vi "PV_DataLog_v2.vi"() -> ()   [LabVIEW 2016]
uses:
  MGCC_DataLog_global.vi
  Global tdms reference.vi
  Communication/Global communication.vi
  <vilib>/Utility/error.llb/Error Cluster From Error Code.vi
  Finite State Machine (He Yin)/Sub-VIs/MGCC_FntStaMach_gobal.vi
  <vilib>/ErrorRing/Error Ring.xnode
panel:
  in  "Start":bool=TRUE
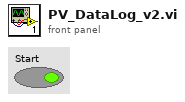
[diagram p1: front panel]
types:
  T1 = enum16{"open", "open or create", "create or replace", "create", "open (read-only)"}
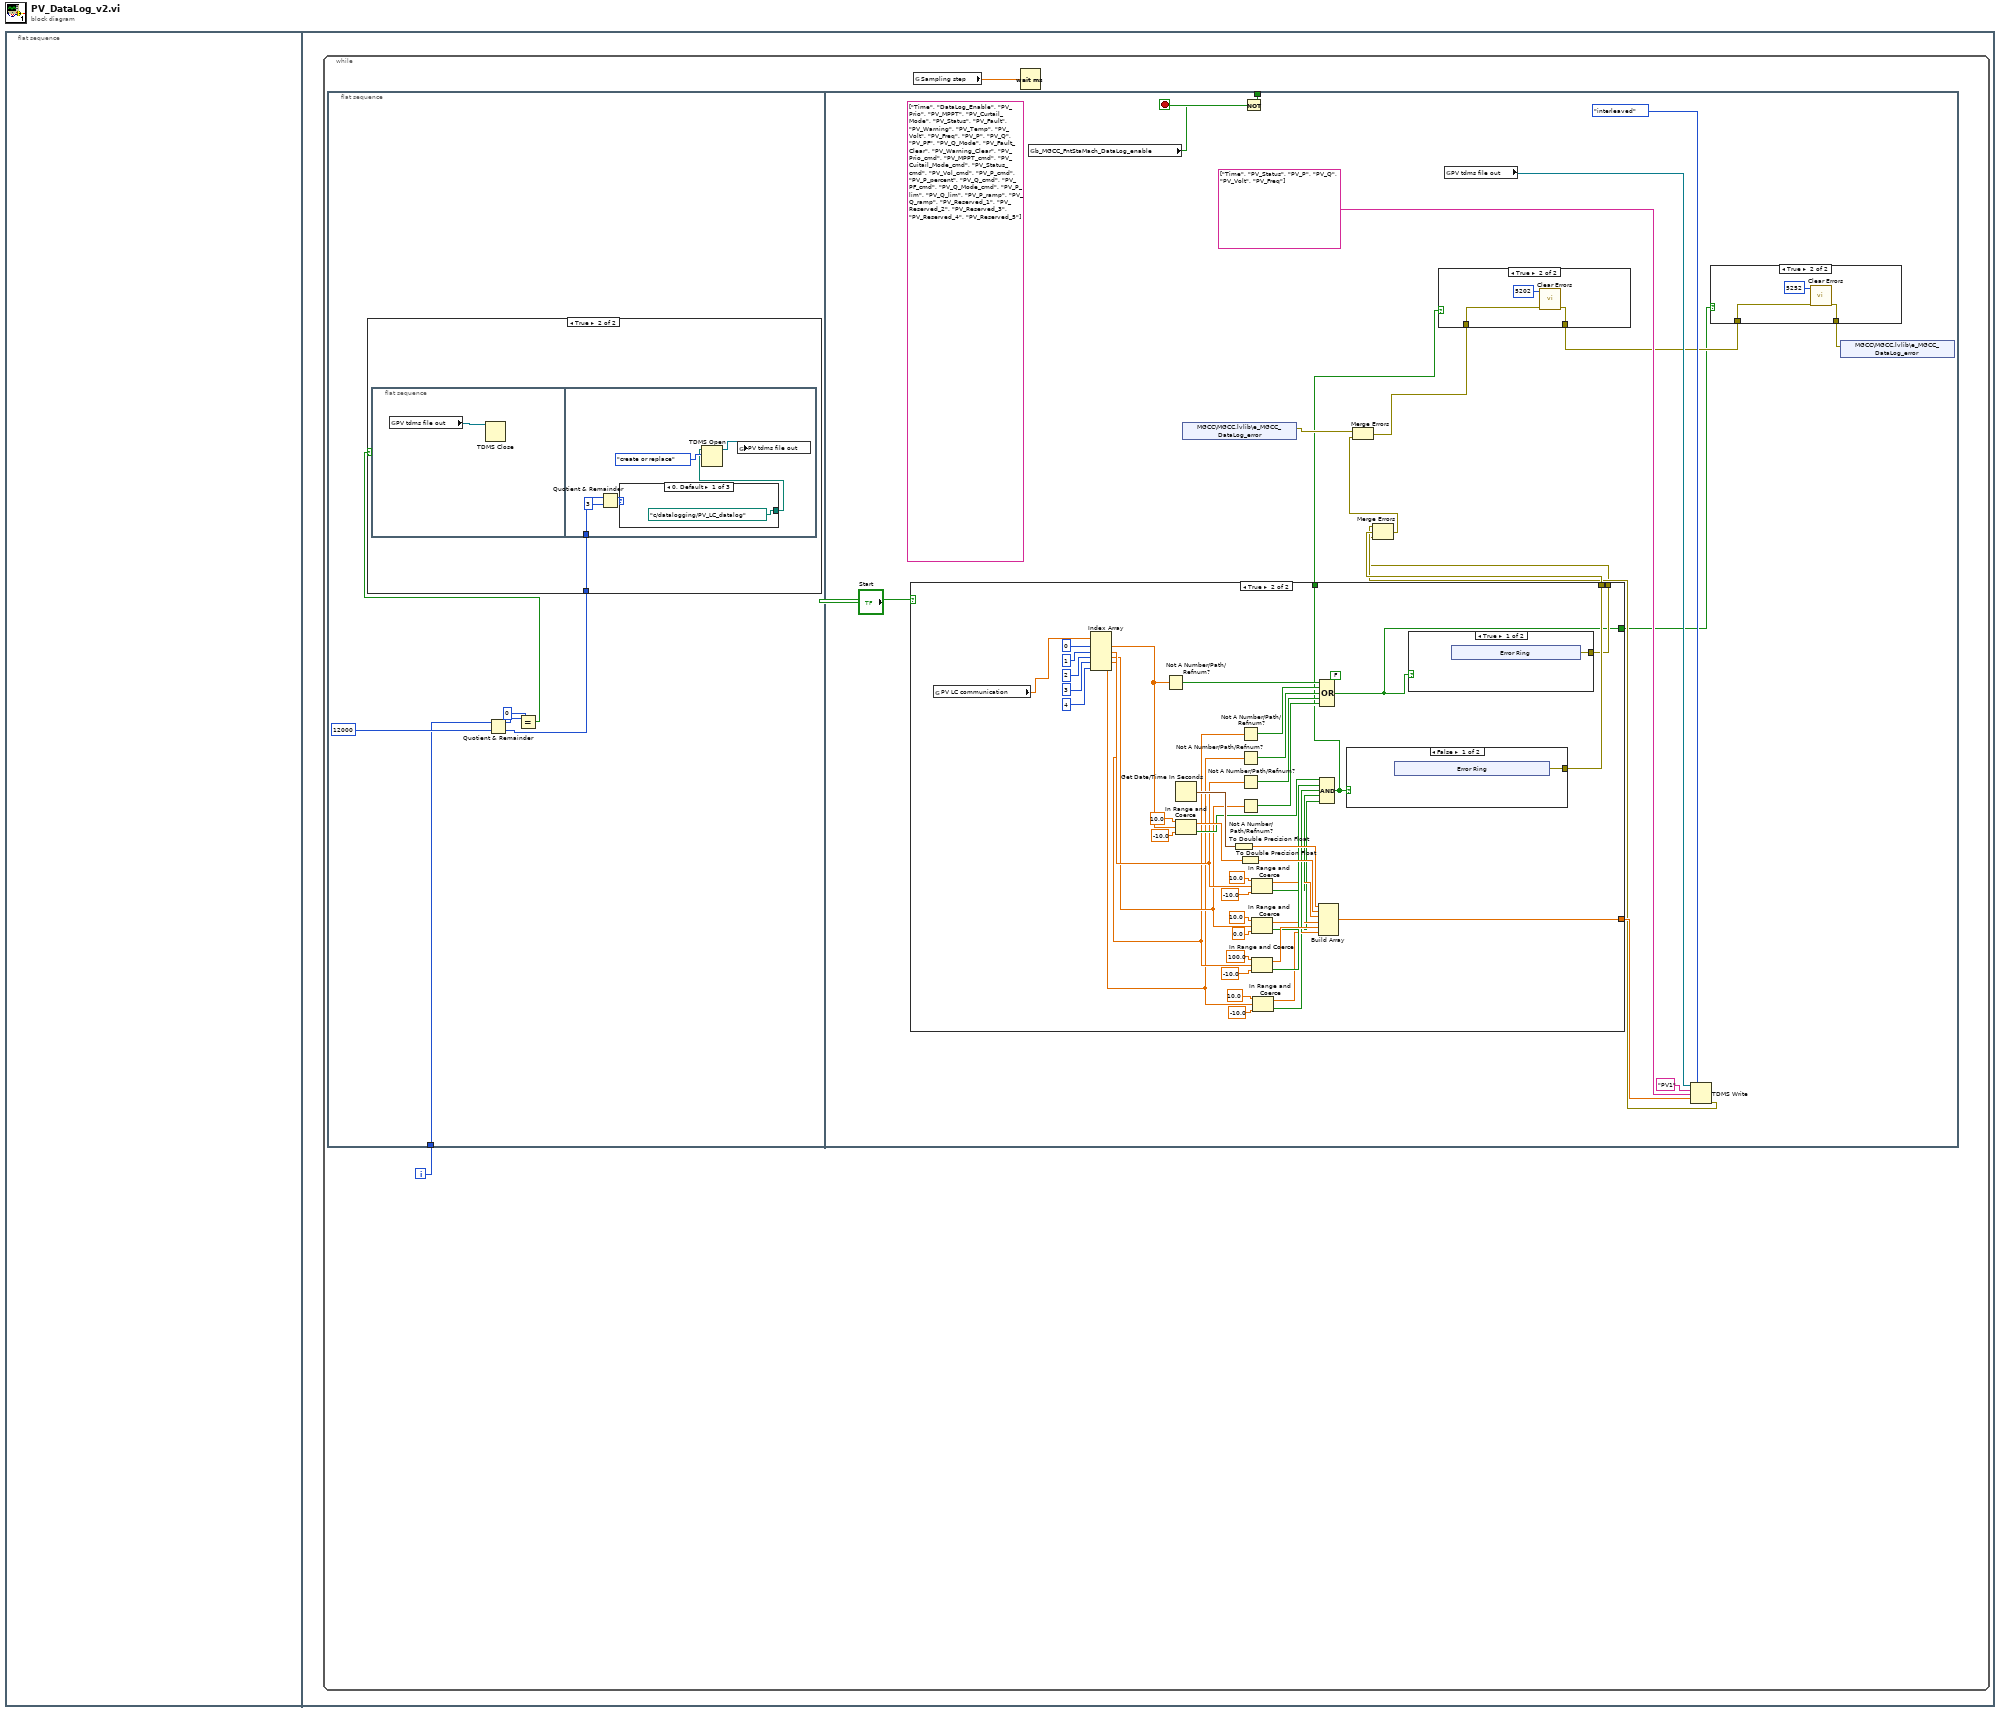
[diagram p0: block diagram]
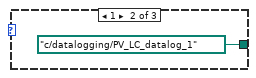
[diagram p3: hidden frame]
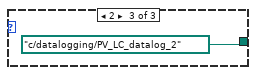
[diagram p4: hidden frame]
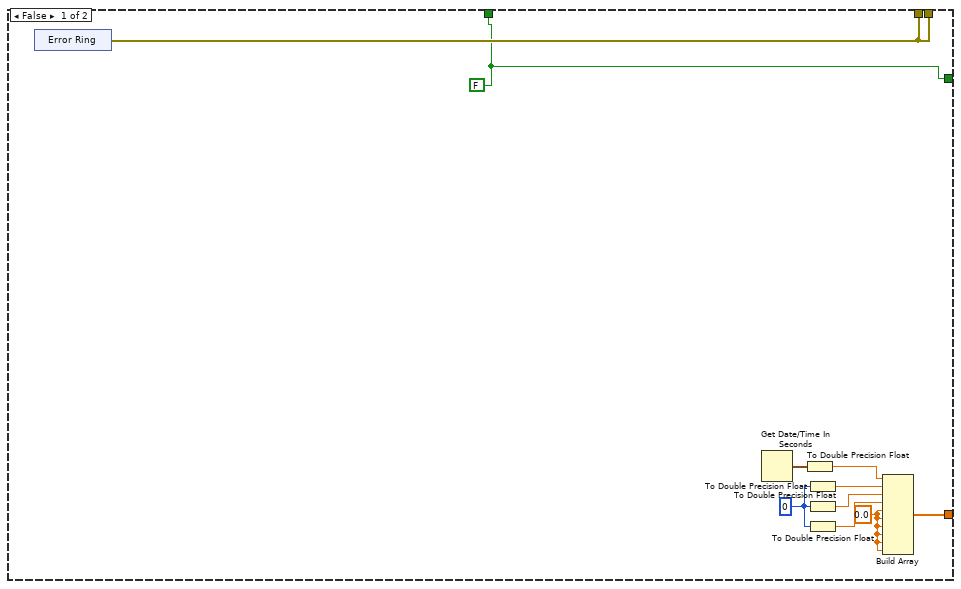
[diagram p7: hidden frame]
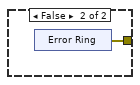
[diagram p8: hidden frame]
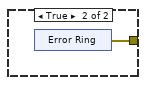
[diagram p9: hidden frame]
diagram:
  n1 = flat-sequence {
    frame #0 {
    }
    frame #1 {
      n2 = while {
        i -> [w1]
        stop <- w3 stop-if-true
        n3 = flat-sequence {
          tunnel: w1 -> [w4]
          tunnel: [w34] -> w3
          frame #0 {
            n4 = Quotient & Remainder(x=w4, y=12000) -> (x-y*floor(x/y)=w8:i32, floor(x/y)=w5:i32)
            n5 = Equal?(x=w8, y=0) -> (x = y?=w6:bool)
            n6 = case shown="True" w6 {
              tunnel: w5 -> [_ w10]
              frame False {
              }
              frame True {
                n7 = flat-sequence {
                  tunnel: w10 -> [w15]
                  frame #0 {
                    n8 = global read "Global tdms reference.vi" "PV tdms file out"() -> (w11:refnum<k34>)
                    n9 = TDMS Close(11:w11) -> ()  [unwired: 1 in, 2 out]
                  }
                  frame #1 {
                    n10 = Quotient & Remainder(x=w15, y=3) -> (x-y*floor(x/y)=w13:i32)  [unwired: 1 out]
                    n11 = case shown="0, Default" w13 {
                      tunnel: [path "c:/datalogging/PV_LC_datalog" ("file path (dialog if empty)") path "c:/datalogging/PV_LC_datalog_1" ("file path (dialog if empty)") path "c:/datalogging/PV_LC_datalog_2" ("file path (dialog if empty)")] -> w12
                      frame 0, Default {
                      }
                      frame 1 {
                      }
                      frame 2 {
                      }
                    }
                    n12 = TDMS Open(10:T1."create or replace" ("operation (0:open)"), 11:w12) -> (3:w17:refnum<k34>)  [unwired: 5 in, 1 out]
                    n13 = global write "Global tdms reference.vi" "PV tdms file out"(w17) -> ()
                  }
                }
              }
            }
          }
          frame #1 {
            (unwired) string[] ["Time", "DataLog_Enable", "PV_Prio", "PV_MPPT", "PV_Curtail_Mode", "PV_Status", "PV_Fault", "PV_Warning", "PV_Temp", "PV_Volt", "PV_Freq", "PV_P", "PV_Q", "PV_PF", "PV_Q_Mode", "PV_Fault_Clear", "PV_Warning_Clear", "PV_Prio_cmd", "PV_MPPT_cmd", "PV_Cuitail_Mode_cmd", "PV_Status_cmd", "PV_Vol_cmd", "PV_P_cmd", "PV_P_percent", "PV_Q_cmd", "PV_PF_cmd", "PV_Q_Mode_cmd", "PV_P_lim", "PV_Q_lim", "PV_P_ramp", "PV_Q_ramp", "PV_Reserved_1", "PV_Reserved_2", "PV_Reserved_3", "PV_Reserved_4", "PV_Reserved_5"] ("channel name(s) in (Untitled)")
            n14 = case shown="True" "Start" {
              tunnel: [w51 w101] -> w36
              tunnel: [w48 w77] -> w31
              tunnel: [w48 w71] -> w28
              tunnel: [w47 w70] -> w26
              tunnel: [w47 w58] -> w22
              frame False {
                w47 = FALSE
                w53 = 0.0
                w50 = 0
                n15 = xnode "Error Ring"() -> ("error out"=w48:errorcluster)
                n16 = Get Date/Time In Seconds() -> (seconds since 1Jan1904=w49:timestamp)
                n17 = To Double Precision Float(number=w49) -> (double precision float=w52:dbl)
                n18 = To Double Precision Float(number=w50) -> (double precision float=w56:dbl)
                n19 = To Double Precision Float(number=w50) -> (double precision float=w55:dbl)
                n20 = To Double Precision Float(number=w50) -> (double precision float=w54:dbl)
                n21 = Build Array(w52, w56, w55, w54, w53, w53, w53, w53, w53, w53) -> (w51:dbl[])
              }
              frame True {
                (unwired) FALSE
                n22 = global read "Global communication.vi" "PV LC communication"() -> (w59:dbl[])
                n23 = Index Array(array=w59, index #1=0 ("index"), index #2=1 ("index"), index #3=2 ("index"), index #4=3 ("index"), index #5=4 ("index")) -> (element #1=w64:dbl, element #2=w63:dbl, element #3=w62:dbl, element #4=w61:dbl, element #5=w60:dbl)
                n24 = Not A Number/Path/Refnum?(number/path/refnum=w64) -> (NaN/Path/Refnum?=w76:bool)
                n25 = Get Date/Time In Seconds() -> (seconds since 1Jan1904=w100:timestamp)
                n26 = In Range and Coerce(upper limit=10.0, x=w64, lower limit=-10.0) -> (coerced(x)=w97:dbl, In Range?=w94:bool)
                n27 = To Double Precision Float(number=w100) -> (double precision float=w99:dbl)
                n28 = Not A Number/Path/Refnum?(number/path/refnum=w61) -> (NaN/Path/Refnum?=w75:bool)
                n29 = Not A Number/Path/Refnum?(number/path/refnum=w60) -> (NaN/Path/Refnum?=w74:bool)
                n30 = Not A Number/Path/Refnum?(number/path/refnum=w63) -> (NaN/Path/Refnum?=w73:bool)
                n31 = Not A Number/Path/Refnum?(number/path/refnum=w62) -> (NaN/Path/Refnum?=w72:bool)
                n32 = To Double Precision Float(number=w97) -> (double precision float=w98:dbl)
                n33 = In Range and Coerce(upper limit=10.0, x=w63, lower limit=-10.0) -> (coerced(x)=w85:dbl, In Range?=w82:bool)
                n34 = In Range and Coerce(upper limit=10.0, x=w62, lower limit=0.0) -> (coerced(x)=w81:dbl, In Range?=w78:bool)
                n35 = In Range and Coerce(upper limit=100.0, x=w61, lower limit=-10.0) -> (coerced(x)=w91:dbl, In Range?=w90:bool)
                n36 = In Range and Coerce(upper limit=10.0, x=w60, lower limit=-10.0) -> (coerced(x)=w87:dbl, In Range?=w86:bool)
                n37 = Build Array(w99, w98, w85, w81, w91, w87) -> (w101:dbl[])
                n38 = Compound Arithmetic op=OR(w76, w75, w74, w73, w72) -> (w58:bool)
                n39 = Compound Arithmetic op=AND(w94, w90, w86, w82, w78) -> (w70:bool)
                n40 = case shown="False" w70 {
                  tunnel: [w110 w116] -> w77
                  frame False {
                    n41 = xnode "Error Ring"() -> ("error out"=w110:errorcluster)
                  }
                  frame True {
                    n42 = xnode "Error Ring"() -> ("error out"=w116:errorcluster)
                  }
                }
                n43 = case shown="True" w58 {
                  tunnel: [w102 w108] -> w71
                  frame True {
                    n44 = xnode "Error Ring"() -> ("error out"=w102:errorcluster)
                  }
                  frame False {
                    n45 = xnode "Error Ring"() -> ("error out"=w108:errorcluster)
                  }
                }
              }
            }
            n46 = global read "MGCC_FntStaMach_gobal.vi" "b_MGCC_FntStaMach_DataLog_enable"() -> (w21:bool)
            n47 = shared-variable "MGCC\\MGCC.lvlib\\e_MGCC_DataLog_error"() -> (w32:errorcluster)  [unwired: 1 in, 1 out]
            n48 = Not(x=w21) -> (.not. x?=w34:bool)
            n49 = global read "Global tdms reference.vi" "PV tdms file out"() -> (w25:refnum<k34>)
            n50 = TDMS Write(0:w25, 1:enum16{"decimated", "interleaved"}."interleaved" ("data layout (0:decimated)"), 5:"PV1" ("group name in (Untitled)"), 7:string[] ["Time", "PV_Status", "PV_P", "PV_Q", "PV_Volt", "PV_Freq"] ("channel name(s) in (Untitled)"), 9:w36) -> (15:w29:errorcluster)  [unwired: 1 in, 3 out]
            n51 = Merge Errors(w29, w31, w28) -> (w30:errorcluster)
            n52 = Merge Errors(w32, w30) -> (w27:errorcluster)
            n53 = case shown="True" w26 {
              tunnel: w27 -> [w43 w46]
              tunnel: [w43 w44] -> w23
              frame False {
              }
              frame True {
                n54 = call <vilib>:"Clear Errors.vi"("error in (no error)"=w46, "specific error code to clear (0: all)"=5202) -> ("error out"=w44:errorcluster)  [unwired: 4 in, 1 out]
              }
            }
            n55 = case shown="True" w22 {
              tunnel: w23 -> [w39 w42]
              tunnel: [w39 w40] -> w24
              frame False {
              }
              frame True {
                n56 = call <vilib>:"Clear Errors.vi"("error in (no error)"=w42, "specific error code to clear (0: all)"=5252) -> ("error out"=w40:errorcluster)  [unwired: 4 in, 1 out]
              }
            }
            n57 = shared-variable "MGCC\\MGCC.lvlib\\e_MGCC_DataLog_error"(w24) -> ()  [unwired: 1 in, 1 out]
          }
        }
        n58 = global read "MGCC_DataLog_global.vi" "Sampling step"() -> (w2:dbl)
        n59 = Wait (ms)(milliseconds to wait=w2) -> ()  [unwired: 1 out]
      }
    }
  }
